vi "From VConfig.vi"(8 "error in (no error)":errorcluster, 10 "Variant":variant, 11 "Modbus TCP Micro Master in":refnum<class "Modbus TCP Micro Master.lvclass">) -> (0 "error out":errorcluster, 3 "Modbus TCP Micro Master out":refnum<class "Modbus TCP Micro Master.lvclass">)   [LabVIEW 2023, in "Modbus TCP Micro.lvlib" / "Modbus TCP Micro Master.lvclass"]
uses:
  Modbus TCP Micro Master.lvclass
  Modbus TCP Micro Master.lvclass/Modbus TCP Micro Master.ctl
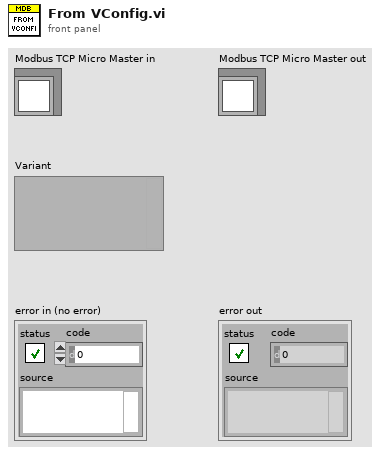
[diagram p1: front panel]
types:
  T1 = typedef "Modbus TCP Micro.lvlib/Modbus TCP Micro Master.lvclass/Settings.ctl" = cluster{"address":string, "remote port or service name":u16, "timeout ms (10000)":i32, "local port (0)":u16}
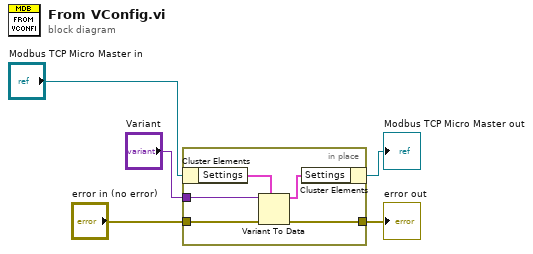
[diagram p0: block diagram]
diagram:
  n1 = in-place {
    in-place-border: "error in (no error)" -> [w10]
    in-place-border: "Variant" -> [w9]
    in-place-border: [w8] -> w1
    n2 = in-place-cluster #1("Modbus TCP Micro Master in") -> ("Settings"=w7:T1)
    n3 = Variant To Data(error in=w10, type=w7, Variant=w9) -> (data=w6:T1, error out=w8:errorcluster)
    n4 = in-place-cluster #1("Settings"=w6) -> (→"Modbus TCP Micro Master out":refnum<class "Modbus TCP Micro Master.lvclass">)
  }
  "error out" <- w1
